vi "fuzzyex Set Move Direction.vi"(1 "direction":bool, 2 "beta":dbl format="%.2f", 3 "y(VC)":dbl format="%.2f", 4 "x(VC)":dbl format="%.2f") -> (0 "New Dir":bool)   [LabVIEW 2023]
doc: "This VI calculates the appropriate moving direction within the vehicle drive control example depending on the vehicle center coordinates, the vehicle orientation angle and the current moving direction. If the vehicle cannot be moved backwards to reach its end position, it is moved forward to get enough space to drive backwards again."
panel:
  # "x-coordinate vehicle center"
  # "Forward driving"
  # "y-coordinate vehicle center"
  # "Backward driving"
  # "vehicle orientation angle"
  # "Forward driving"
  # "Backward driving"
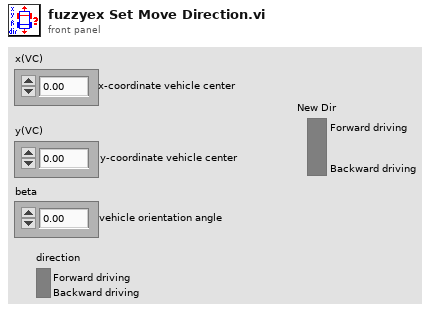
[diagram p1: front panel]
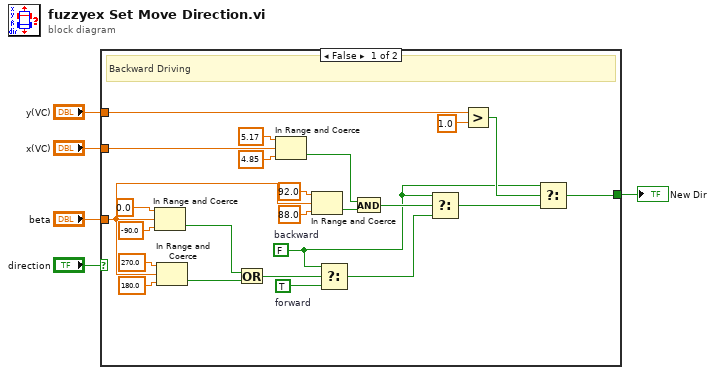
[diagram p0: block diagram]
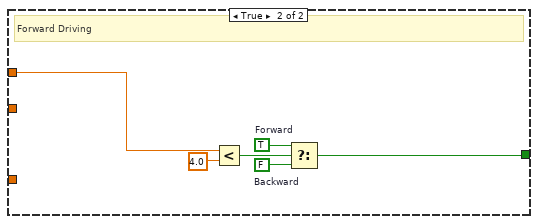
[diagram p2: hidden frame]
diagram:
  n1 = case shown="False" "direction" {
    tunnel: "x(VC)" -> [w27 _]
    tunnel: "y(VC)" -> [w8 w35]
    tunnel: "beta" -> [w13 _]
    tunnel: [w19 w30] -> w1
    frame False {
      w6 = FALSE  # backward
      w9 = TRUE  # forward
      # "Backward Driving"
      n2 = In Range and Coerce(upper limit=0.0, x=w13, lower limit=-90.0) -> (In Range?=w12:bool)  [unwired: 1 out]
      n3 = In Range and Coerce(upper limit=270.0, x=w13, lower limit=180.0) -> (In Range?=w11:bool)  [unwired: 1 out]
      n4 = Or(x=w12, y=w11) -> (x .or. y?=w7:bool)
      n5 = In Range and Coerce(upper limit=5.17, x=w27, lower limit=4.85) -> (In Range?=w22:bool)  [unwired: 1 out]
      n6 = In Range and Coerce(upper limit=92.0, x=w13, lower limit=88.0) -> (In Range?=w18:bool)  [unwired: 1 out]
      n7 = Select(t=w6, s=w7, f=w9) -> (s? t:f=w10:bool)
      n8 = And(x=w22, y=w18) -> (x .and. y?=w21:bool)
      n9 = Select(t=w6, s=w21, f=w10) -> (s? t:f=w20:bool)
      n10 = Greater?(x=w8, y=1.0) -> (0:w28:bool)
      n11 = Select(t=w6, s=w28, f=w20) -> (s? t:f=w19:bool)
    }
    frame True {
      w31 = FALSE  # Backward
      w32 = TRUE  # Forward
      # "Forward Driving"
      n12 = Less?(x=w35, y=4.0) -> (x < y?=w33:bool)
      n13 = Select(t=w32, s=w33, f=w31) -> (s? t:f=w30:bool)
    }
  }
  "New Dir" <- w1
